vi "Motor driver 10 to 1 v9.0.2.vi"() -> ()   [LabVIEW 2009]
panel:
  in  "Resource Name":refnum<visa-resource-name>="ASRL1::INSTR"
  out "current command":ext=0.014850395057373172892 format="%.6f"
  out "current set pt":ext=0.0115343950573731728925 format="%.6f"
  in  "# of pts":u16(ring) items=["3", "5", "10", "20"]
  out "?":ext(graph)=0.005367
  out "?":dbl(graph)=0.02
  in  "smooth":bool=TRUE
  out "Motor running":bool
  in  "Withdraw piston":T1={"withdrawal rate"=enum."-8E-05 \"/s"}
  in  "OK":bool
  out "Sent string":string="S "
  in  "Mode":i32(listbox)=2
  out "current reset":ext=0.5493019999999999999 format="%.6f"
  in  "initial reset":ext=0.1 format="%.2f"
  out "local var: load first time flag":bool
  out "internal force gauge (v)":ext=0.004623333333333333333 format="%.6f"
  in  "Constant load":T2={"set pt"=0.012, "Int"=0.00099999999999999999996, "Prop"=20000.0, "hi reset limit"=1.0, "total limit"=0.02, "gauge zero"=0.003316, "1st pist contact (V)"=0.91740000000000000003, "lo reset limit"=0.0} {"lo reset limit" format="%.6f"; "1st pist contact (V)" format="%.4f"; "gauge zero" format="%.6f"; "total limit" format="%.2f"; "hi reset limit" format="%.6f"; "Prop" format="%.2f"; "Int" format="%.6f"; "set pt" format="%.6f"}
  in  "Constant displacement rate":T3={"displacement rate"=enum."8E-05 \"/s"}
  in  "Load relaxation":cluster{"Does absolutely nothing":u8, bool}
  in  "stop/go":bool
  out "Active string":string="S "
  out "Read String":string="S "
  out "current selected displacement rate":string
  # "Note: Correct \"Resource Name may be\ndynamic.  If error or if no function, try\ndifferent resources in the pull-down list."
  # "^SEE NOTE"
  # "Constant load only. \"Mode\" menu disabled"
  # "Just push the STOP buttom, dummy"
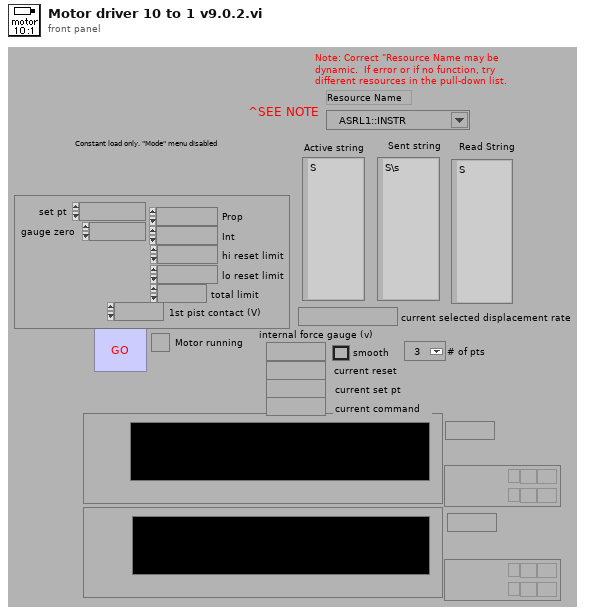
[diagram p1: front panel]
types:
  T1 = cluster{"withdrawal rate":enum16{"-8E-04 \"/s", "-8E-07 \"/s", "-8E-06 \"/s", "-8E-05 \"/s"}}
  T2 = cluster{"set pt":ext, "Int":ext, "Prop":ext, "hi reset limit":ext, "total limit":ext, "gauge zero":ext, "1st pist contact (V)":ext, "lo reset limit":ext}
  T3 = cluster{"displacement rate":enum16{"8E-04 \"/s", "8E-07 \"/s", "8E-06 \"/s", "8E-05 \"/s"}}
  T4 = enum16{"-8E-04 \"/s", "-8E-07 \"/s", "-8E-06 \"/s", "-8E-05 \"/s"}
  T5 = enum16{"8E-04 \"/s", "8E-07 \"/s", "8E-06 \"/s", "8E-05 \"/s"}
  T6 = cluster{ext, "Int":ext, "Prop":ext, "hi reset limit":ext, "total limit":ext, "lo reset limit":ext}
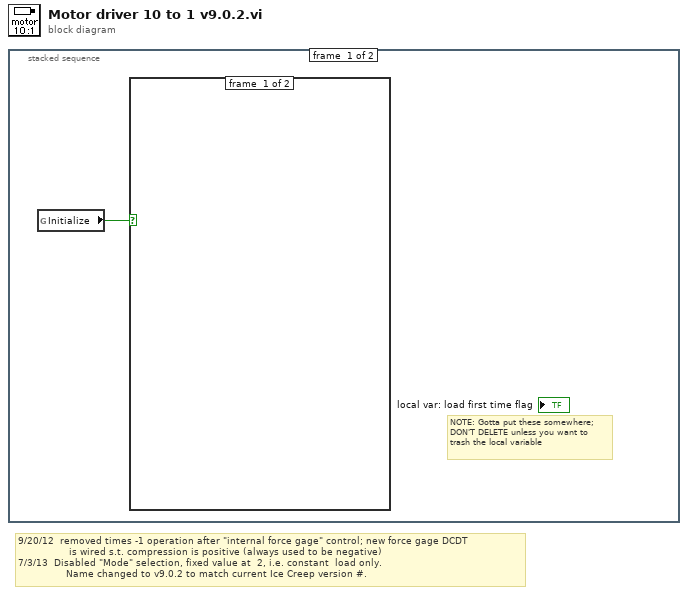
[diagram p0: block diagram]
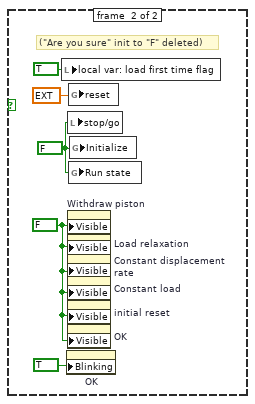
[diagram p2: hidden frame]
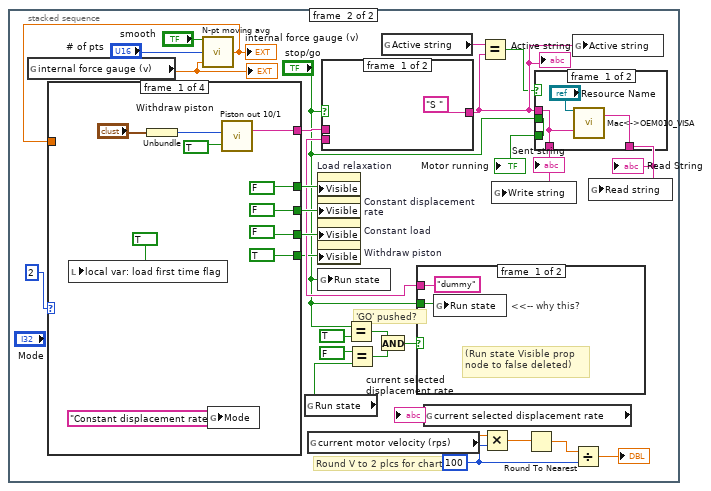
[diagram p3: hidden frame]
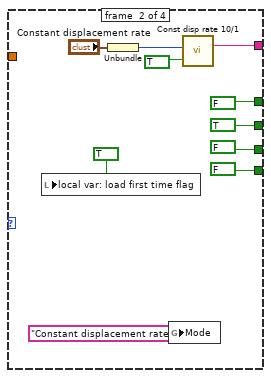
[diagram p5: hidden frame]
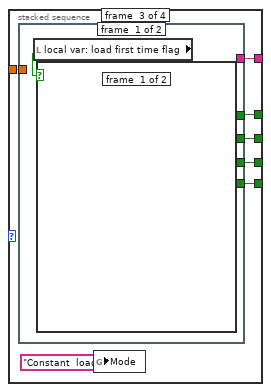
[diagram p6: hidden frame]
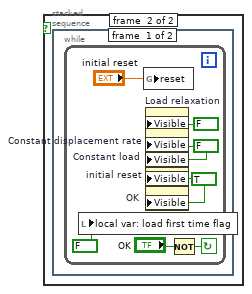
[diagram p7: hidden frame]
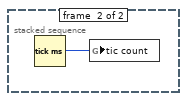
[diagram p8: hidden frame]
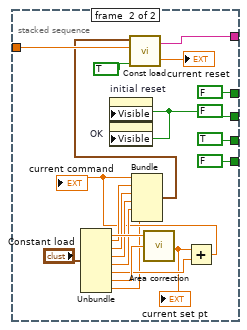
[diagram p9: hidden frame]
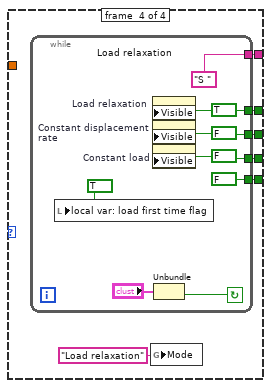
[diagram p10: hidden frame]
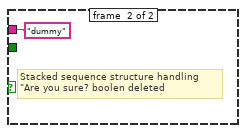
[diagram p11: hidden frame]
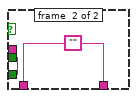
[diagram p12: hidden frame]
diagram:
  # "9/20/12  removed times -1 operation after \"internal force gage\" control; new force gage DCDT\n                 is wired s.t. compression is positive (always used to be negative)\n7/3/13  Disabled \"Mode\" selection, fixed value at  2, i.e. constant  load only.\n                Name changed to v9.0.2 to match current Ice Creep version #."
  n1 = stacked-sequence {
    frame #0 {
      # "NOTE: Gotta put these somewhere; DON'T DELETE unless you want to trash the local variable"
      n2 = global read "Motor drive globals" "Initialize"() -> (w1:bool)
      n3 = case shown="True" w1 {
        frame #0 {
        }
        frame #1 {
          w4 = FALSE
          w2 = FALSE
          # "(\"Are you sure\" init to \"F\" deleted)"
          n4 = local write "local var: load first time flag"(TRUE) -> ()
          n5 = property on="OK" class="Boolean"("Blinking"=TRUE) -> ()  [unwired: 2 in, 2 out]
          n6 = local write "stop/go"(w4) -> ()
          n7 = property on="Withdraw piston" class="Cluster (strict)"("Visible"=w2) -> ()  [unwired: 2 in, 2 out]
          n8 = property on="Load relaxation" class="Cluster"("Visible"=w2) -> ()  [unwired: 2 in, 2 out]
          n9 = property on="Constant displacement rate" class="Cluster (strict)"("Visible"=w2) -> ()  [unwired: 2 in, 2 out]
          n10 = property on="Constant load" class="Clust (strict)"("Visible"=w2) -> ()  [unwired: 2 in, 2 out]
          n11 = property on="initial reset" class="Digital (strict)"("Visible"=w2) -> ()  [unwired: 2 in, 2 out]
          n12 = property on="OK" class="Boolean"("Visible"=w2) -> ()  [unwired: 2 in, 2 out]
          n13 = global write "Motor drive globals" "reset"(ext 0.0) -> ()
          n14 = global write "Motor drive globals" "Run state"(w4) -> ()
          n15 = global write "Motor drive globals" "Initialize"(w4) -> ()
        }
      }
    }
    frame #1 {
      w13 = 100
      # "Round V to 2 plcs for chart"
      # "'GO' pushed?"
      n16 = global read "Motor drive globals" "internal force gauge (v)"() -> (w8:ext)
      "?" <- w8
      n17 = call "N-pt moving avg"("Current input vaue"=w8, "# of pts"="# of pts", "Smooth"="smooth") -> ("Moving average"=w14:ext)
      "internal force gauge (v)" <- w14
      n18 = case shown="3.." 2 {
        tunnel: [w44 w53 w62 w97] -> w30
        tunnel: [FALSE FALSE w65 w100] -> w31
        tunnel: [FALSE TRUE w64 w99] -> w32
        tunnel: [FALSE FALSE w63 w98] -> w33
        tunnel: [TRUE FALSE w60 w95] -> w20
        tunnel: w14 -> [_ _ w59 _]
        frame #0 {
          n19 = local write "local var: load first time flag"(TRUE) -> ()
          n20 = Unbundle("Withdraw piston") -> ("withdrawal rate"=w48:T4)
          n21 = global write "Motor drive globals" "Mode"("Constant displacement rate") -> ()
          n22 = call "Piston out 10/1"("Start"=TRUE, "withdrawal rate"=w48) -> ("Write String"=w44:string)  [unwired: 1 in]
        }
        frame #1 {
          n23 = local write "local var: load first time flag"(TRUE) -> ()
          n24 = Unbundle("Constant displacement rate") -> ("displacement rate"=w57:T5)
          n25 = global write "Motor drive globals" "Mode"("Constant displacement rate") -> ()
          n26 = call "Const disp rate 10/1"("Start"=TRUE, "displacement rate"=w57) -> ("Write String"=w53:string)  [unwired: 1 in]
        }
        frame #2 {
          n27 = stacked-sequence {
            tunnel: [_ FALSE] -> w65
            tunnel: [_ w89] -> w64
            tunnel: [_ TRUE] -> w63
            tunnel: [_ w90] -> w62
            tunnel: [_ FALSE] -> w60
            tunnel: w59 -> [_ w87]
            frame #0 {
              n28 = local read "local var: load first time flag"() -> (w66:bool)
              n29 = case shown="True" w66 {
                frame #0 {
                }
                frame #1 {
                  n30 = stacked-sequence {
                    frame #0 {
                      n31 = while {
                        stop <- w68 continue-if-true
                        w73 = FALSE
                        w67 = TRUE
                        n32 = local write "local var: load first time flag"(FALSE) -> ()
                        n33 = global write "Motor drive globals" "reset"("initial reset") -> ()
                        n34 = property on="Load relaxation" class="Cluster"("Visible"=FALSE) -> ()  [unwired: 2 in, 2 out]
                        n35 = property on="Constant displacement rate" class="Cluster (strict)"("Visible"=w73) -> ()  [unwired: 2 in, 2 out]
                        n36 = property on="Constant load" class="Clust (strict)"("Visible"=w73) -> ()  [unwired: 2 in, 2 out]
                        n37 = property on="initial reset" class="Digital (strict)"("Visible"=w67) -> ()  [unwired: 2 in, 2 out]
                        n38 = property on="OK" class="Boolean"("Visible"=w67) -> ()  [unwired: 2 in, 2 out]
                        n39 = Not(x="OK") -> (.not. x?=w68:bool)
                      }
                    }
                    frame #1 {
                      n40 = Tick Count (ms)() -> (millisecond timer value=w74:u32)
                      n41 = global write "Motor drive globals" "tic count"(w74) -> ()
                    }
                  }
                }
              }
            }
            frame #1 {
              w89 = FALSE
              n42 = Unbundle("Constant load") -> ("set pt"=w85:ext, "Int"=w83:ext, "Prop"=w82:ext, "hi reset limit"=w81:ext, "total limit"=w80:ext, "gauge zero"=w79:ext, "1st pist contact (V)"=w84:ext, "lo reset limit"=w75:ext)
              n43 = property on="initial reset" class="Digital (strict)"("Visible"=w89) -> ()  [unwired: 2 in, 2 out]
              n44 = property on="OK" class="Boolean"("Visible"=w89) -> ()  [unwired: 2 in, 2 out]
              n45 = call "Area correction"("First piston contact (V)"=w84, "Original set point"=w85) -> ("Current set point"=w76:ext)  [unwired: 1 out]
              "current set pt" <- w76
              n46 = Add(x=w76, y=w79) -> (x+y=w77:ext)
              "current command" <- w77
              n47 = Bundle(w77, "Int"=w83, "Prop"=w82, "hi reset limit"=w81, "total limit"=w80, "lo reset limit"=w75) -> (w78:T6)  [unwired: 1 in]
              n48 = call "Const load"("send values"=TRUE, "internal force guage (v)"=w87, 5:w78) -> ("current reset"=→"current reset":ext, "Write String"=w90:string)  [unwired: 1 in]
            }
          }
          n49 = global write "Motor drive globals" "Mode"("Constant  load") -> ()
        }
        frame #3 {
          n50 = while {
            tunnel: [w107] -> w100
            tunnel: [w106] -> w99
            tunnel: [w105] -> w98
            tunnel: ["S "] -> w97
            tunnel: [FALSE] -> w95
            stop <- w102 continue-if-true
            w107 = TRUE
            w106 = FALSE
            w105 = FALSE
            n51 = local write "local var: load first time flag"(TRUE) -> ()
            n52 = property on="Load relaxation" class="Cluster"("Visible"=w107) -> ()  [unwired: 2 in, 2 out]
            n53 = property on="Constant displacement rate" class="Cluster (strict)"("Visible"=w106) -> ()  [unwired: 2 in, 2 out]
            n54 = property on="Constant load" class="Clust (strict)"("Visible"=w105) -> ()  [unwired: 2 in, 2 out]
            n55 = Unbundle("Load relaxation") -> (w102:bool)  [unwired: 1 out]
          }
          n56 = global write "Motor drive globals" "Mode"("Load relaxation") -> ()
        }
      }
      n57 = global read "Motor drive globals" "Run state"() -> (w19:bool)
      n58 = global read "Motor drive globals" "current motor velocity (rps)"() -> (w12:dbl)
      n59 = property on="Load relaxation" class="Cluster"("Visible"=w31) -> ()  [unwired: 2 in, 2 out]
      n60 = property on="Constant displacement rate" class="Cluster (strict)"("Visible"=w32) -> ()  [unwired: 2 in, 2 out]
      n61 = property on="Constant load" class="Clust (strict)"("Visible"=w33) -> ()  [unwired: 2 in, 2 out]
      n62 = property on="Withdraw piston" class="Cluster (strict)"("Visible"=w20) -> ()  [unwired: 2 in, 2 out]
      n63 = global write "Motor drive globals" "Run state"("stop/go") -> ()
      n64 = Equal?(x="stop/go", y=TRUE) -> (x = y?=w23:bool)
      n65 = Equal?(x=FALSE, y=w19) -> (x = y?=w22:bool)
      n66 = And(x=w23, y=w22) -> (x .and. y?=w26:bool)
      n67 = global read "Motor drive globals" "Active string"() -> (w36:string)
      n68 = case shown="True" w26 {
        tunnel: ["dummy" "dummy"] -> w21
        tunnel: "stop/go" -> [w109 _]
        frame #0 {
          # "(Run state Visible prop node to false deleted)"
          # "<<-- why this?"
          n69 = global write "Motor drive globals" "Run state"(w109) -> ()
        }
        frame #1 {
          # "Stacked sequence structure handling \"Are you sure? boolen deleted"
        }
      }
      n70 = case shown="True" "stop/go" {
        tunnel: w30 -> [_ w38]
        tunnel: w21 -> [_ _]
        tunnel: ["S " w38] -> w35
        frame #0 {
        }
        frame #1 {
          # "T/F reacting to \"Are you sure\" boolean deleted."
        }
      }
      "Active string" <- w35
      n71 = global read "Motor drive globals" "current selected displacement rate"() -> (→"current selected displacement rate":string)
      n72 = Equal?(x=w36, y=w35) -> (x = y?=w34:bool)
      n73 = Multiply(x=w12, y=w13) -> (x*y=w9:dbl)
      n74 = Round To Nearest(number=w9) -> (nearest integer value=w10:dbl)
      n75 = case shown="False" w34 {
        tunnel: w35 -> [w113 _]
        tunnel: [w114 w117] -> w28
        tunnel: [w113 w117] -> w27
        tunnel: [w115 w116] -> w18
        tunnel: "stop/go" -> [w115 w116]
        frame #0 {
          n76 = call "Mac<->OEM010_VISA"("Resource Name"="Resource Name", "Serial Write"=w113) -> ("Serial Read"=w114:string)  [unwired: 12 in, 5 out]
        }
        frame #1 {
          w117 = ""
        }
      }
      "Read String" <- w28
      "Sent string" <- w27
      "Motor running" <- w18
      n77 = global write "Motor drive globals" "Write string"(w27) -> ()
      n78 = global write "Motor drive globals" "Active string"(w35) -> ()
      n79 = Divide(x=w10, y=w13) -> (x/y=→"?":dbl)
      n80 = global write "Motor drive globals" "Read string"(w28) -> ()
    }
  }
